vi "setup_R_configurations.vi"(11 "Resistances":dbl[](array[numeric])) -> (3 "configs":cluster{dbl, bool[]}[](array[cluster]))   [LabVIEW 2018]
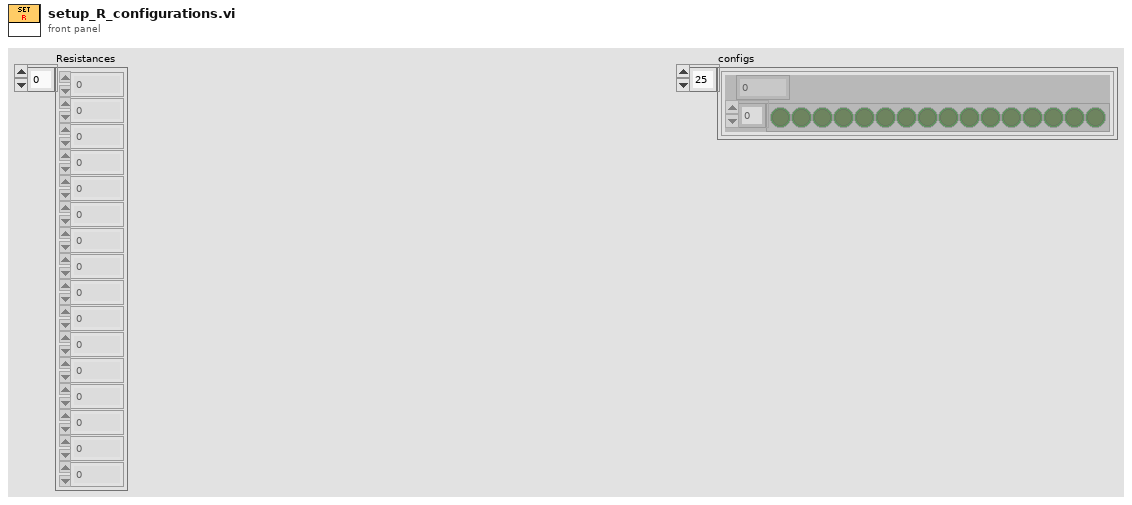
[diagram p1: front panel]
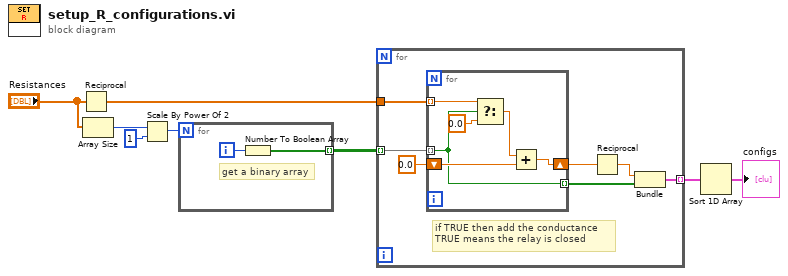
[diagram p0: block diagram]
diagram:
  n1 = Reciprocal(x="Resistances") -> (1/x=w7:dbl[])
  n2 = Array Size(array="Resistances") -> (size(s)=w4:i32)
  n3 = Scale By Power Of 2(n=w4, x=1 ("nr of resistors")) -> (x*2^n=w5:i32)
  n4 = for {
    N: w5 -> [_]
    tunnel: [w9] -> w3 mode=indexing
    i -> [w10]
    # "get a binary array"
    n5 = Number To Boolean Array(number=w10) -> (Boolean array=w9:bool[])
  }
  n6 = for {
    tunnel: w3 -> [w17] mode=indexing
    tunnel: w7 -> [w16]
    tunnel: [w13] -> w2 mode=indexing
    # "if TRUE then add the conductance\nTRUE means the relay is closed"
    n7 = for {
      tunnel: w17 -> [w18] mode=indexing
      tunnel: w16 -> [w23] mode=indexing
      shift-right: [w19] -> w12
      shift-left: 0.0 -> [w20]
      tunnel: [w18] -> w14 mode=indexing
      n8 = Select(t=w23, s=w18, f=0.0 ("cas faux")) -> (s? t:f=w21:dbl)
      n9 = Add(x=w21, y=w20) -> (x+y=w19:dbl)
    }
    n10 = Reciprocal(x=w12) -> (1/x=w11:dbl)
    n11 = Bundle(w11, w14) -> (w13:cluster{dbl, bool[]})  [unwired: 1 in]
  }
  n12 = Sort 1D Array(array=w2) -> (sorted array=→"configs":cluster{dbl, bool[]}[])
